vi "CommonSig-Tone Burst Channel.vi"(0 "Name":string, 7 "Destination":string) -> (8 "Channel out":refnum<class "Channel.lvclass">)   [LabVIEW 2020]
uses:
  Classes/Channel/Channel.lvclass
  Classes/Channel/Channel.lvclass/Channel.ctl
  Classes/Channel/Write Waveform.vi
  Classes/Channel/Write Gate.vi
  Classes/Channel/Write Level.vi
  Classes/Channel/Write Destination.vi
  Classes/Waveforms/Tone/Tone.lvclass
  D:/Development/epl-vi-lib/Signal Synthesis VIs/4th Generation/Classes/Waveforms/Waveform/Waveform.lvclass
  Classes/Level/Level.lvclass
  Classes/Gate/Gate.lvclass
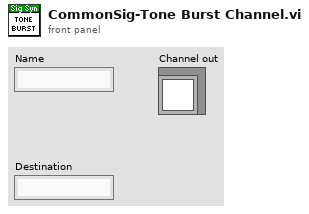
[diagram p1: front panel]
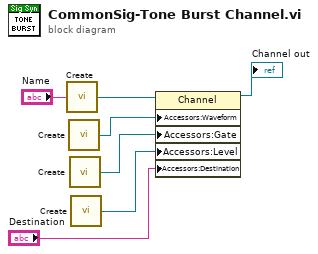
[diagram p0: block diagram]
diagram:
  n1 = call "Create.vi"("Name"="Name") -> ("Channel"=w2:refnum<class "Channel.lvclass">)  [unwired: 14 in]
  n2 = call "Create.vi"() -> ("Tone"=w4:refnum<class "Tone.lvclass">)  [unwired: 15 in]
  n3 = call "Create.vi"() -> ("Gate"=w5:refnum<class "Gate.lvclass">)  [unwired: 15 in]
  n4 = call "Create.vi"() -> ("Level"=w6:refnum<class "Level.lvclass">)  [unwired: 15 in]
  n5 = property class="Channel"(reference=w2, "Accessors:Waveform"=w4, "Accessors:Gate"=w5, "Accessors:Level"=w6, "Accessors:Destination"="Destination") -> (reference out=→"Channel out":refnum<class "Channel.lvclass">)  [unwired: 1 in, 1 out]
